vi "RT - Write Config.vi"(8 "error in":errorcluster, 11 "PARAMETERS":T1={"Body CalPara"={"Slope"=62500.0, "Intercept"=-250.0}, "US CalPara"={"Slope"=62500.0, "Intercept"=-250.0}} {"US CalPara"."Intercept" format="%.6f"; "US CalPara"."Slope" format="%.6f"; "Body CalPara"."Intercept" format="%.6f"; "Body CalPara"."Slope" format="%.6f"}) -> (0 "error out":errorcluster)   [LabVIEW 2018]
uses:
  Controls/Parameters.ctl
  Controls/Sensor CalPara.ctl
  Controls/ConfigData.ctl
  Controls/ConfigString.ctl
  Globals/Global - Configuration Options.vi
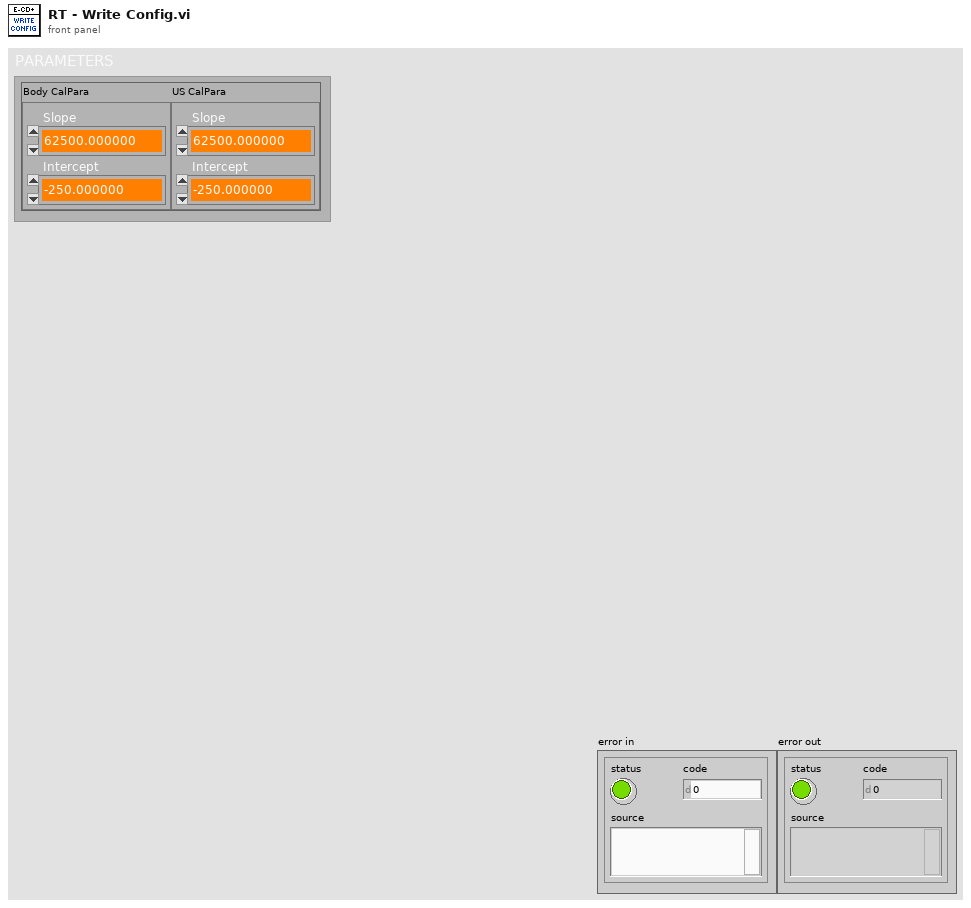
[diagram p1: front panel]
types:
  T1 = typedef "Parameters.ctl" = cluster{"Body CalPara":T2, "US CalPara":T2}
  T2 = typedef "Sensor CalPara.ctl" = cluster{"Slope":dbl, "Intercept":dbl}
  T3 = typedef "ConfigString.ctl" = cluster{"BODY CAL":string[], "US CAL":string[]}
  T4 = typedef "ConfigData.ctl" = cluster{"BODY CAL":dbl[], "US CAL":dbl[]}
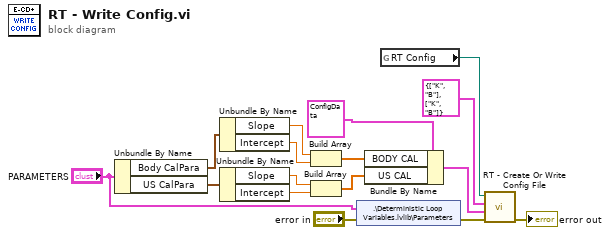
[diagram p0: block diagram]
diagram:
  n1 = Unbundle By Name("PARAMETERS") -> ("Body CalPara"=w13:T2, "US CalPara"=w12:T2)
  n2 = Unbundle By Name(w13) -> ("Slope"=w15:dbl, "Intercept"=w14:dbl)
  n3 = Unbundle By Name(w12) -> ("Slope"=w5:dbl, "Intercept"=w4:dbl)
  n4 = Build Array(w15, w14) -> (w6:dbl[])
  n5 = Build Array(w5, w4) -> (w2:dbl[])
  n6 = shared-variable ".\\Deterministic Loop Variables.lvlib\\Parameters"("PARAMETERS", error in="error in") -> (error out=w10:errorcluster)
  n7 = Bundle By Name(cluster=T4 {"BODY CAL"=[468750.0, -1875.0], "US CAL"=[468750.0, -1875.0]} ("CONFIG DATA"), "BODY CAL"=w6, "US CAL"=w2) -> (w8:T4)
  n8 = global read "Global - Configuration Options.vi" "RT Config"() -> (w11:path)
  n9 = call "RT - Create Or Write Config File.vi"("error in"=w10, "CONFIG DATA"=w8, "CONFIG STRING"=T3 {"BODY CAL"=["K", "B"], "US CAL"=["K", "B"]}, "ConfigFile Path In"=w11) -> ("error out"=→"error out":errorcluster)  [unwired: 6 in, 1 out]
